vi "1111_#NoPidoFile.vi"(6 "Kp":dbl, 7 "error":dbl, 9 "Offset":dbl, 10 "Limit in":dbl, 11 "Thresh":dbl) -> (2 "Limit out":dbl, 3 "Boolean":bool)   [LabVIEW 2014]
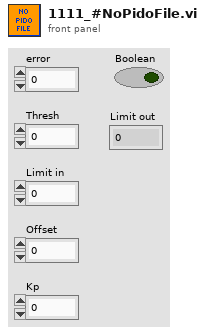
[diagram p1: front panel]
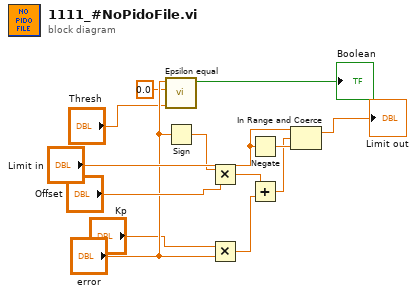
[diagram p0: block diagram]
diagram:
  n1 = call "Epsilon equal.vi"("Epsilon"="Thresh", "Value2"=0.0 ("Epsilon"), "Value1"="error") -> ("Boolean"=→"Boolean":bool)  [unwired: 8 in]
  n2 = Sign(1:"error") -> (0:w8:dbl)
  n3 = Multiply(x=w8, y="Offset") -> (x*y=w9:dbl)
  n4 = Multiply(x="Kp", y="error") -> (x*y=w4:dbl)
  n5 = Negate(x="Limit in") -> (-x=w13:dbl)
  n6 = Add(x=w9, y=w4) -> (x+y=w10:dbl)
  n7 = In Range and Coerce(upper limit="Limit in", x=w10, lower limit=w13) -> (coerced(x)=→"Limit out":dbl)  [unwired: 1 out]
